vi "Is Changed.vi"(11 "Config Element in":refnum<class "Config Element.lvclass">) -> (2 "Changed":bool)   [LabVIEW 2020, in "CDM-Config.lvlib" / "Config Element.lvclass"]
uses:
  Config Element.lvclass
  Config Element.lvclass/Config Element.ctl
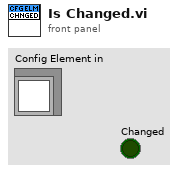
[diagram p1: front panel]
types:
  T1 = typedef "CDM-Config.lvlib/Config Element.lvclass/Ref Data.ctl" = cluster{"Config Element":T2, "Node Info":T4, "Owner":refnum<class>, "Changed":bool}
  T2 = typedef "CDM-Config.lvlib/Config Element.ctl" = cluster{"Hierarchy":string[], "Value":string, "Meta Data":T3[]}
  T3 = typedef "CDM-Config.lvlib/Meta Data.ctl" = cluster{"Name":string, "Value":string}
  T4 = typedef "CDM-Config.lvlib/Node Info.ctl" = cluster{"Index":i32, "Parent":i32, "Children":i32[]}
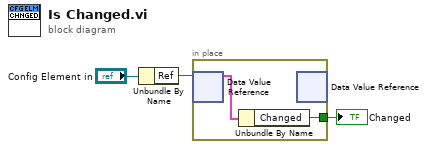
[diagram p0: block diagram]
diagram:
  n1 = Unbundle By Name("Config Element in") -> ("Ref"=w3:refnum<data-value>)
  n2 = in-place {
    in-place-border: [w4] -> w1
    n3 = in-place-dvr #1(w3) -> (w5:T1)  [unwired: 1 out]
    n4 = Unbundle By Name(w5) -> ("Changed"=w4:bool)
    n5 = in-place-dvr #1() -> ()  [unwired: 1 in, 2 out]
  }
  "Changed" <- w1
